vi "Parse State Queue++.vi"(0 "State Queue":string, 1 "Name (\"\" to Use UUID)":string, 2 "Response Arguments":string, 7 "Previous Error":errorcluster, 9 "Dequeue (1 ms)":i32=1, 11 "Response Timeout (-2 Use Global Settings)":i32=-2, 12 "Allowed Messages (Empty for All)":string[](array[string])) -> (3 "Name Used":string, 4 "Remaining States":string, 6 "Current State":string, 8 "Arguments":string, 10 ">> Response Source Message >>":T1, 15 ">> Source CSM >>":string)   [LabVIEW 2017, in "Communicable State Machine.lvlib"]
doc: "### Parse State Queue++.vi\n\nParses the CSM state queue and returns the next current state to be executed, along with parameters and other information.\n\n<b>Controls</b>\n- <b>State Queue</b>: The entire state queue is connected to this input. This should come from the CSM's shift register.\n- <b>Previous Error</b>: The error cluster from the CSM is connected to this input. If an error occurs and appears at this input, the current state output will return the \"Error Handler\" state.\n- <b>Name (\"\" to use uuid)</b>: CSM module name.\n- <b>Response Timeout(-2 using Global Settings)</b>: Response timeout setting for synchronous calls, If -2 is specified, the global setting will be used. You can use \"CSM - Set TMO of Sync-Reply.vi\" to change the global setting.\n- <b>Dequeue Timeout (0ms)</b>: Timeout setting for checking the CSM message queue, default is 0, meaning no wait.\n- <b>Response Arguments</b>: Response parameters from the previous state. It should be connected to the CSM's shift register to pass return values from external calls.\n\n<b>Indicators</b>\n- <b>Remaining States</b>: All concatenated states and parameters.\n- <b>Arguments</b>: Returns any parameters that may be used in the current state string. These parameters are located after the \">>\" character. <b>Note:</b> Argument variables must not contain any non-printable characters, such as newline or carriage return.\n- <b>Current State</b>: The next current state to be executed.\n- <b>Name Used</b>: The actual name assigned to this CSM module.\n- <b>Argument - State</b>: If it is a built-in state defined by CSM, this parameter indicates the previous state of this state.\n- <b>From Who</b>: If <b>Current State</b> is sent by an external source, this is the source CSM module name."
uses:
  Communicable State Machine.lvlib
  _Support/Typedef/_CSM_Response Source Message.ctl
  _Support/Typedef/_CSM_GlobalLog_MSG.ctl
  _Support/Typedef/_CSM_GlobalLog_MSG_TYPE.ctl
  _Support/Typedef/_CSM_MSG_TYPE.ctl
  _Support/Typedef/_CSM Status Change Event Data.ctl
  _Support/CSMQ/_CSMObj-Message Check.vi
  _Support/CSMQ/_CSMObj-Enqueue Cross-Module Message.vi
  _Support/CSMQ/_CSMOFGV Get.vi
  _Support/GlobalEvent/GEvt-Generate with Rule Check.vi
  _Support/FGV-BroadcastRegistry/Cache-Broadcast Registry Search Result.vi
  _Support/Common/Hex Str to U8 Data.vi
  AdvanceAPI/CSM - Revert Arguments-Safe String.vi
  AdvanceAPI/CSM - Make String Arguments Safe.vi
  _Support/Common/U8 Data to Hex Str.vi
  _Support/Priority Queue/Dequeue Element.vi
  _Support/GlobalEvent/GEvt-Convert Filter Rules - v1.0.vi
  _Support/ChangeFlag/FlagInstance-GEvt Filter.vi
  _Shared/CSM - System States.vi
  _Support/Priority Queue/Enqueue Element.vi
  _Support/ChangeFlag/FlagInstance-CSMQ FGV.vi
  _Support/ChangeFlag/FlagInstance-Broadcast Cache.vi
  AdvanceAPI/CSM - Keywords.vi
  _Support/ChangeFlag/ChangeFlag-Read.vi
  _Support/GlobalEvent/LogFilter/LogFilter - Check.vi
  _Support/CSMQ/_CSMOFGV(lvlibp).vi
  _Support/FGV-BroadcastRegistry/FGV-BroadcastRegistry(lvlibp).vi
  AdvanceAPI/CSM - List Modules.vi
  _Support/BroadcastRegistry/HelperVI/Broadcast Item Key.vi
  _Shared/Trim Single-line Text.vi
  _Support/ChangeFlag/ChangeFlagDB.vi
  _Support/CSMKVMap/CSMKVMap-Read.vi
  _Support/Error/CSM Not Allowed Message.vi
  _Support/CSMQ/_CSMObj-Add Internal Registry Rule.vi
  _Support/Message/Parse Unregister Message.vi
  _Support/Message/Parse Register Message.vi
  _Shared/Concatenate State with Arguments.vi
  _Support/Error/CSM Missing Return State Error.vi
  Utility/Build Internal State String.vi
  _Shared/Concatenate PostPostMsg Message.vi
  _Support/GlobalEvent/LogFilter/SettingVIs/Set CSM StateType Filter.vi
  _Support/GlobalEvent/LogFilter/SettingVIs/Set Global StateType Filter.vi
  _Support/GlobalEvent/LogFilter/SettingVIs/Set CSM State Filter.vi
  _Support/GlobalEvent/LogFilter/SettingVIs/Set CSM LogType Filter.vi
  _Support/GlobalEvent/LogFilter/SettingVIs/Set Global State Filter.vi
  _Support/GlobalEvent/LogFilter/SettingVIs/Set Global LogType Filter.vi
  _Support/GlobalEvent/LogFilter/SettingVIs/Set Global CSM Filter.vi
  _Support/GlobalEvent/FGV-GEvt Filter Rules(lvlibp).vi
  _Support/GlobalEvent/LogFilter/LogFilter.lvclass
  _Shared/CSM Shared.lvlib
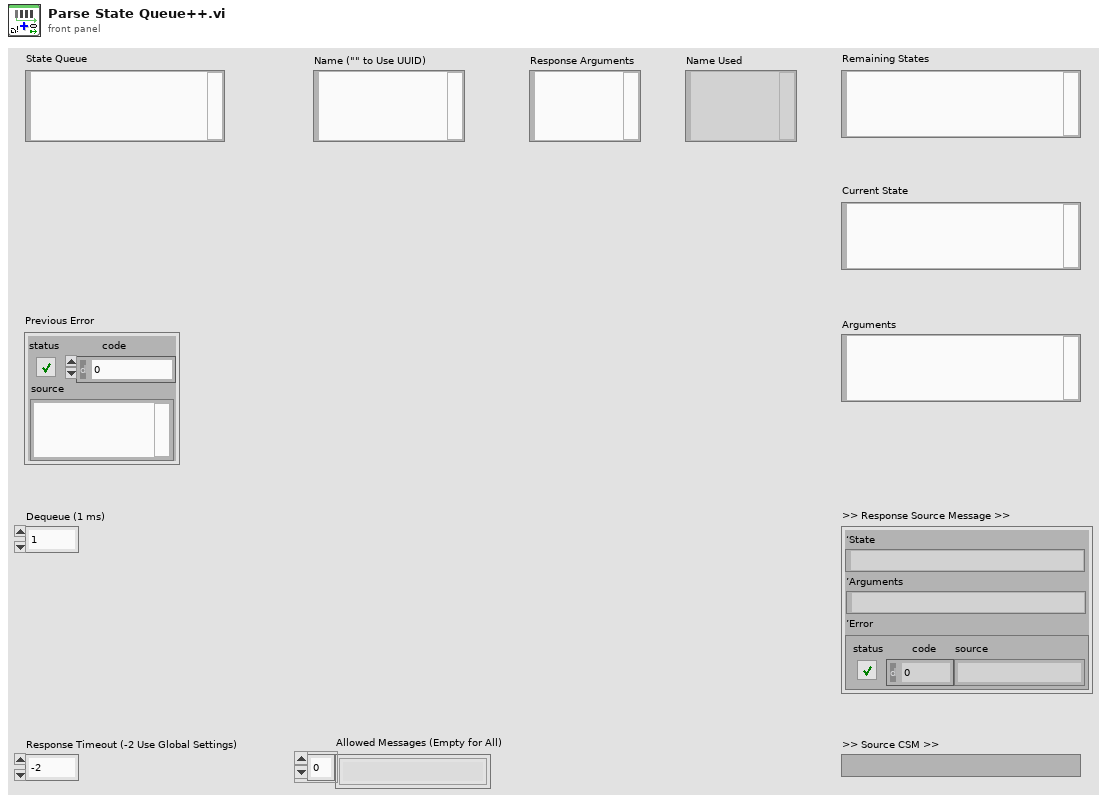
[diagram p1: front panel]
types:
  T1 = typedef "Communicable State Machine.lvlib/_CSM_Response Source Message.ctl" = cluster{"‘State":string, "’Arguments":string, "’Error":errorcluster}
  T2 = typedef "Communicable State Machine.lvlib/_CSM_GlobalLog_MSG.ctl" = cluster{"Name (\"\" to Use UUID)":string, "Current State":string, "Arguments":string, "Source Message":T1, "Source Module":string, "Complete(T)/Start(F)":bool, "LogType":T3, "Time Stamp":timestamp}
  T3 = typedef "Communicable State Machine.lvlib/_CSM_GlobalLog_MSG_TYPE.ctl" = enum16{"User Log", "State Change", "Status", "Interrupt", "Register", "Unregister", "Error Log", "Module Created", "Module Destroyed"}
  T4 = typedef "Communicable State Machine.lvlib/GEvt-Refs.ctl" = cluster{"Event":refnum<user-event>, "Queues":refnum<queue>[], "Valid":bool}
  T5 = typedef "Communicable State Machine.lvlib/_CSMObj.ctl" = cluster{"info":T6, "Refs":T8}
  T6 = typedef "Communicable State Machine.lvlib/_CSMObj-Info.ctl" = cluster{"Module Name":string, "Requested Name":string, "Group Name":string, "Mode":T7, "Allowed Messages":string[]}
  T7 = typedef "Communicable State Machine.lvlib/_CSM_MODE.ctl" = enum16{"Not Exist", "Stand Alone", "CSM", "Worker", "Worker Agent", "Chain Node", "Chain"}
  T8 = typedef "Communicable State Machine.lvlib/_CSMObj-Refs.ctl" = cluster{"WatchDogQ":refnum<queue>, "CSMDataDVR":refnum<data-value>, "Queue":T9, "GroupDataDVR":refnum<data-value>, "TagMap":refnum<data-value>, "ExitEvent":refnum<user-event>, "NewStateEvent":refnum<user-event>, "StatusChangeEvent":refnum<user-event>}
  T9 = typedef "Communicable State Machine.lvlib/Priority Queue.ctl" = cluster{"HPriorityQ":refnum<queue>, "LowPriorityQ":refnum<queue>}
  T10 = typedef "Communicable State Machine.lvlib/_CSM_MSG_TYPE.ctl" = enum16{"Sync Message(-@)", "Async Message(->)", "Async without Response(->|)", "Async Response", "Broadcast(-><all>)", "Broadcast(-><status>)", "Broadcast(-><interrupt>)", "Append to JKISM States", "Append to JKISM States(High Priority)", "Broadcast(-><state>)"}
  T11 = typedef "Communicable State Machine.lvlib/_CSM Status Change Event Data.ctl" = cluster{"ModuleName":string, "Status":string, "Arguments":string}
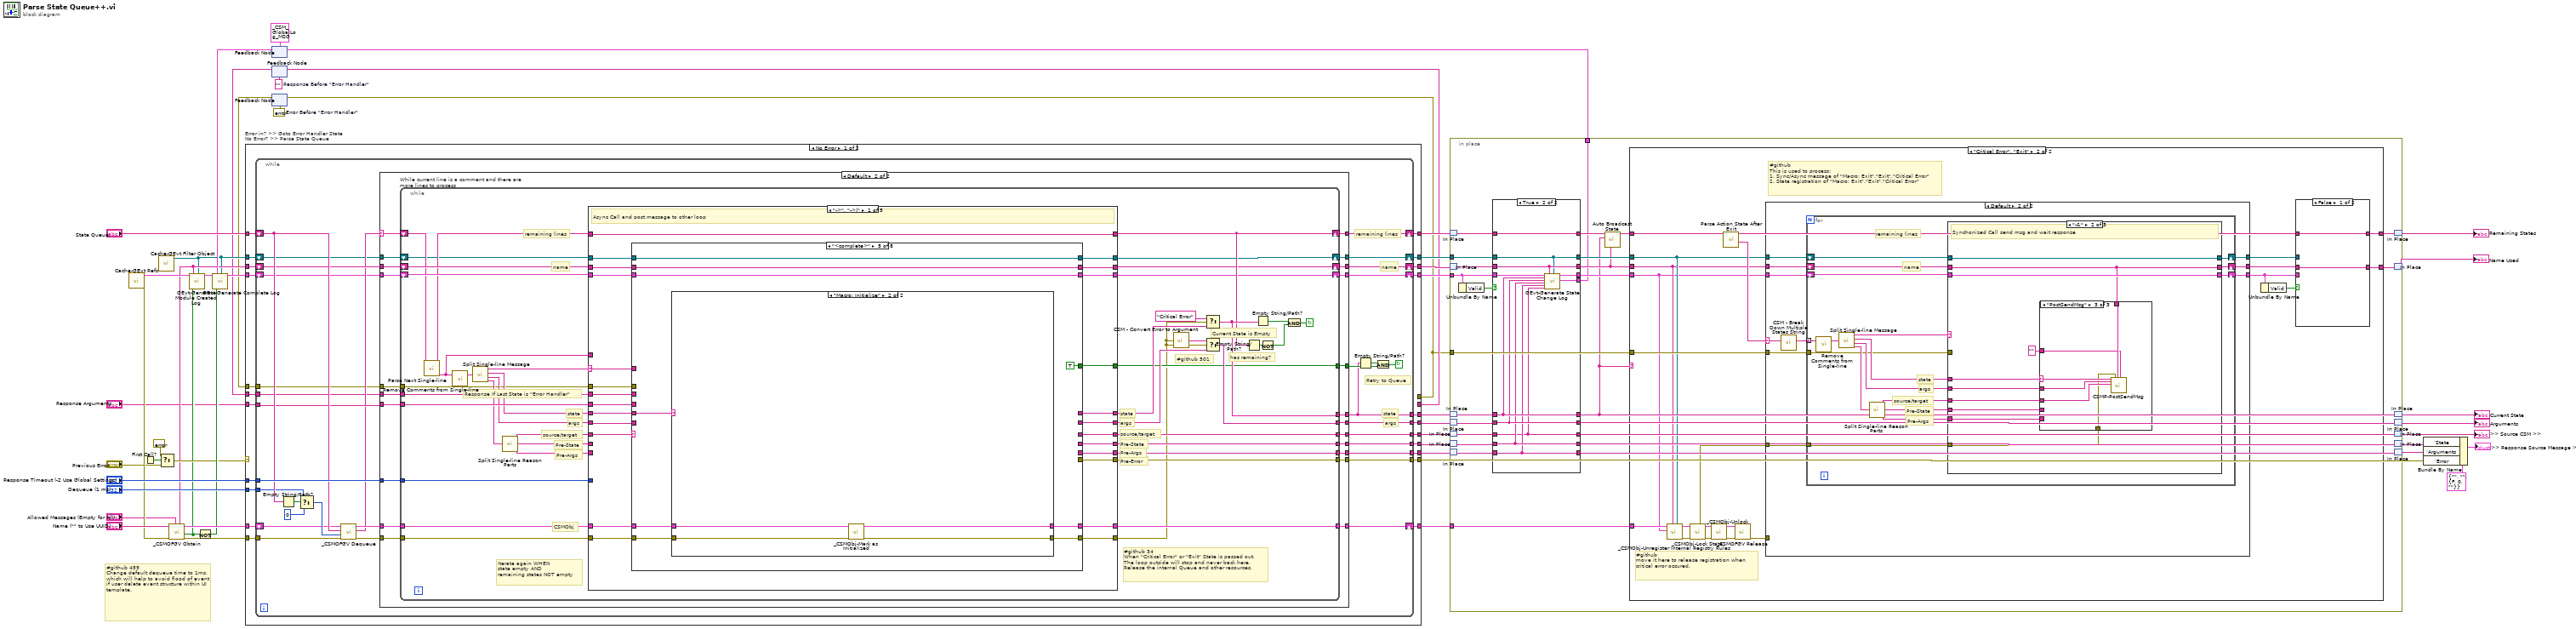
[diagram p0: block diagram]
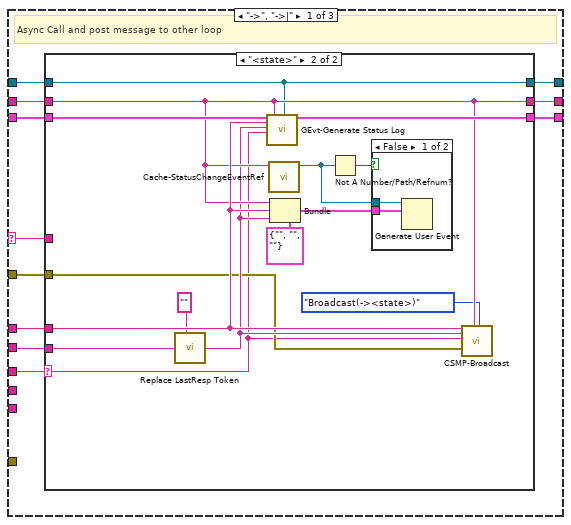
[diagram p4: hidden frame]
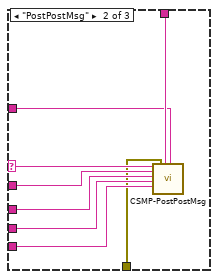
[diagram p8: hidden frame]
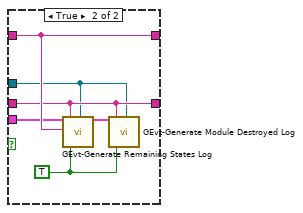
[diagram p10: hidden frame]
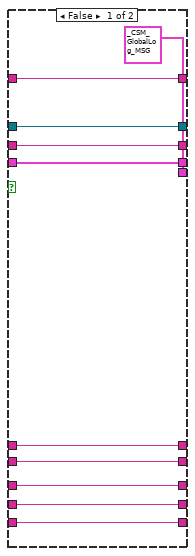
[diagram p11: hidden frame]
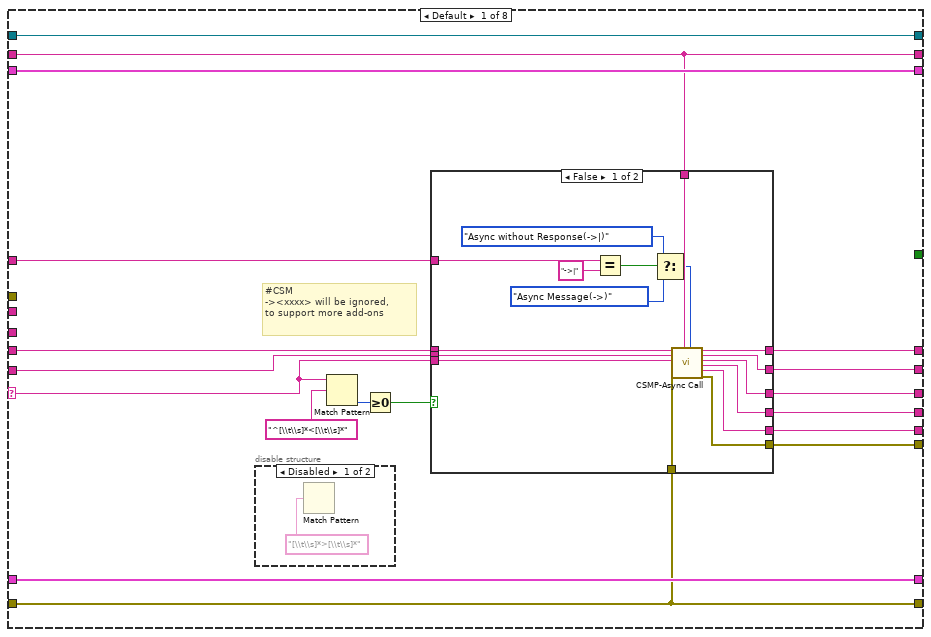
[diagram p13: hidden frame]
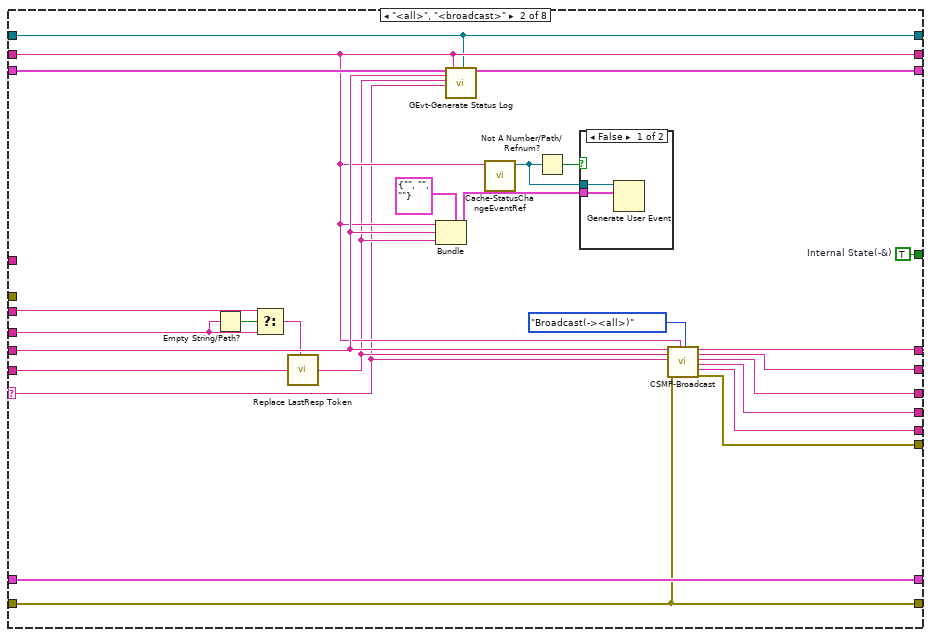
[diagram p16: hidden frame]
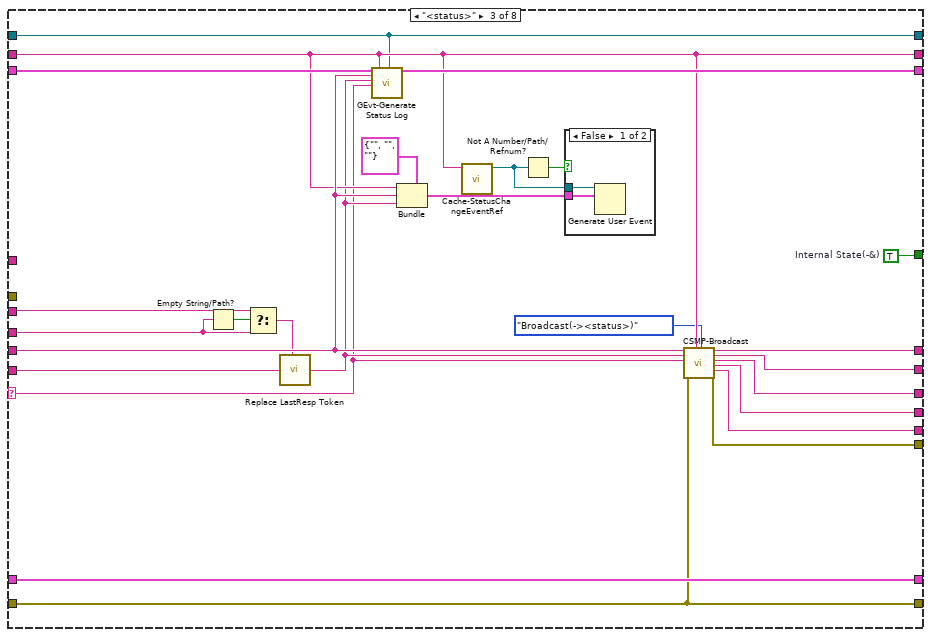
[diagram p18: hidden frame]
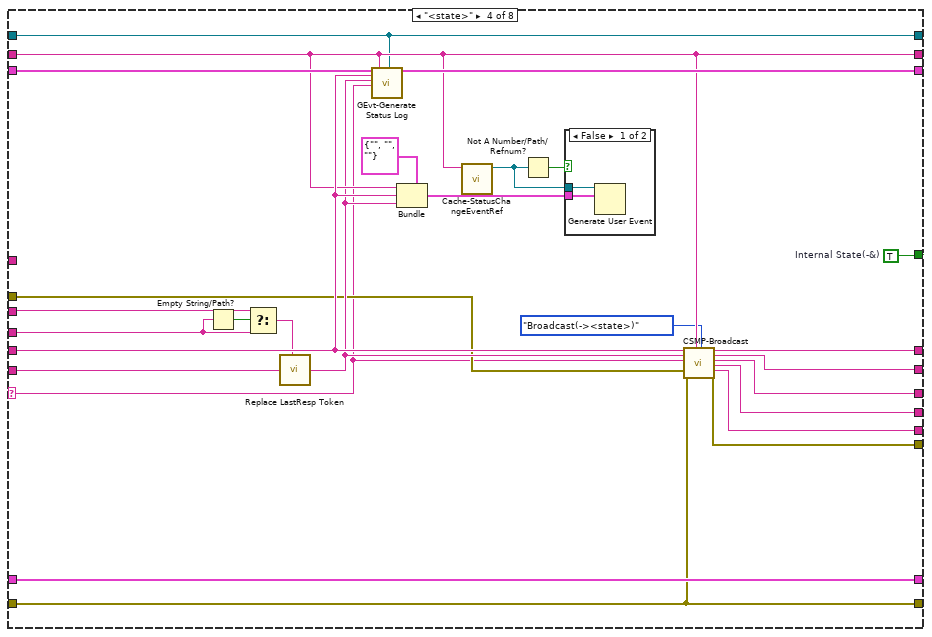
[diagram p20: hidden frame]
diagram:
  w4 = errorcluster {"status"=FALSE, "code"=0, "source"=""}  # Error Before "Error Handler"
  w7 = ""  # Response Before "Error Handler"
  # "#github 459\nChange default dequeue time to 1ms, which will help to avoid flood of event\nif user delete event structure within UI template."
  n1 = call "Cache-GEvt Refs.vi"() -> ("error out"=w33:errorcluster, "CSM Global Log Ref"=w14:T4)  [unwired: 10 in]
  n2 = First Call?() -> (First Call?: T/F=w18:bool)
  n3 = call "Cache-GEvt Filter Object.vi"() -> ("CSM:LogFilter.lvclass"=w9:refnum<class "LogFilter.lvclass">)  [unwired: 11 in]
  n4 = Select(t=errorcluster {"status"=FALSE, "code"=0, "source"=""}, s=w18, f="Previous Error") -> (s? t:f=w16:errorcluster)
  n5 = call "_CSMOFGV Obtain.vi"("Allowed Messages (Empty For All)"="Allowed Messages (Empty for All)", "Error In"=w33, "Name (\"\" to Use UUID) In"="Name (\"\" to Use UUID)") -> ("error out"=w46:errorcluster, "Create? (T)/Cached(F)"=w11:bool, "CSM-Obj"=w45:T5, "Name"=w12:string)  [unwired: 5 in]
  n6 = call "GEvt-Generate Module Created Log.vi"("CSM Global Log Event"=w14, "Name (\"\" to Use UUID)"=w12, "Created?"=w11, "CSM:LogFilter.lvclass"=w9) -> ("CSM Global Log Event Out"=w13:T4)  [unwired: 14 in, 1 out]
  n7 = Not(x=w11) -> (.not. x?=w19:bool)
  n8 = feedback #1(T2 {"Name (\"\" to Use UUID)"="", "Current State"="", "Arguments"="", "Source Message"={"‘State"="", "’Arguments"="", "’Error"={"status"=FALSE, "code"=0, "source"=""}}, "Source Module"="", "Complete(T)/Start(F)"=FALSE, "LogType"=enum."State Change", "Time Stamp"=timestamp(0 s since 1904-01-01)} ("event data")) -> (w24:T2)
  n9 = call "GEvt-Generate Complete Log.vi"("CSM Global Log Event"=w13, "Event Data"=w24, "Enable?"=w19, "CSM:LogFilter.lvclass"=w9) -> ("CSM Global Log Event Out"=w23:T4)  [unwired: 15 in]
  n10 = feedback #2(w7) -> (w5:string)
  n11 = feedback #3(w4) -> (w3:errorcluster)
  n12 = case "Error in? >> Goto Error Handler State\nNo Error? >> Parse State Queue" shown="No Error" w16 {
    selector: w16 -> [_ w582]
    tunnel: [w69 w591] -> w36
    tunnel: [w71 "Error Handler"] -> w44
    tunnel: [w70 w587] -> w43
    tunnel: "State Queue" -> [w66 w591]
    tunnel: "Response Timeout (-2 Use Global Settings)" -> [w68 _]
    tunnel: w45 -> [w61 w586]
    tunnel: [w67 _] -> w41
    tunnel: "Dequeue (1 ms)" -> [w65 _]
    tunnel: [w64 _] -> w42
    tunnel: "Response Arguments" -> [w63 w583]
    tunnel: w46 -> [w62 w585]
    tunnel: w12 -> [w60 w589]
    tunnel: w23 -> [w59 w588]
    tunnel: [w58 w589] -> w32
    tunnel: [w57 w588] -> w31
    tunnel: [w56 _] -> w27
    tunnel: [w55 _] -> w21
    tunnel: w9 -> [w54 w584]
    tunnel: [w53 w584] -> w10
    tunnel: [_ w583] -> w6
    tunnel: w5 -> [w52 _]
    tunnel: [_ w582] -> w2
    tunnel: w3 -> [w51 _]
    tunnel: [w50 w581] -> w1
    frame No Error {
      n13 = while {
        tunnel: [w102] -> w70
        tunnel: w68 -> [w100]
        tunnel: [w99] -> w67
        tunnel: w65 -> [w95]
        tunnel: w62 -> [w90]
        shift-right: [w101] -> w69
        shift-left: w66 -> [w96]
        tunnel: w63 -> [w91]
        tunnel: [w83] -> w71
        tunnel: [w92] -> w64
        shift-right: [w80] -> w58
        shift-left: w60 -> [w88]
        shift-right: [w79] -> w57
        shift-left: w59 -> [w81]
        tunnel: [w78] -> w56
        tunnel: [w77] -> w55
        shift-right: [w75] -> w53
        shift-left: w54 -> [w76]
        tunnel: w52 -> [w74]
        tunnel: w51 -> [w73]
        shift-right: [w72] -> w50
        shift-left: w61 -> [w89]
        stop <- w85 continue-if-true
        # "args"
        # "state"
        # "name"
        # "remaining lines"
        # "Retry to Queue"
        n14 = Empty String/Path?(string/path=w96) -> (empty?=w97:bool)
        n15 = Select(t=w95, s=w97, f=0) -> (s? t:f=w93:i32)
        n16 = call "_CSMOFGV Dequeue.vi"("Error In"=w90, "Dequeue Timeout (0ms)"=w93, "State (S) In (\"\")"=w96, "CSMQ In"=w89) -> ("error out"=w86:errorcluster, "States Out"=w87:string, "CSMQ Out"=w98:T5)  [unwired: 5 in]
        n17 = case shown="Default" w87 {
          selector: w87 -> [_ w122]
          tunnel: [_ w128] -> w83
          tunnel: [_ w127] -> w102
          tunnel: [_ w126] -> w101
          tunnel: w100 -> [_ w125]
          tunnel: [_ w124] -> w99
          tunnel: w88 -> [w106 w123]
          tunnel: w98 -> [w103 w121]
          tunnel: w86 -> [_ w120]
          tunnel: [_ w119] -> w92
          tunnel: w91 -> [_ w118]
          tunnel: [_ w117] -> w84
          tunnel: w81 -> [w105 w116]
          tunnel: [w106 w115] -> w80
          tunnel: [w105 w114] -> w79
          tunnel: [_ w113] -> w78
          tunnel: [_ w112] -> w77
          tunnel: w76 -> [w104 w111]
          tunnel: [w104 w110] -> w75
          tunnel: w74 -> [_ w109]
          tunnel: w73 -> [_ w108]
          tunnel: [w103 w107] -> w72
          frame "" {
            # "Dispatch Mode\n1. Error will Occurred\n2. Add Macro: Exit\n3. The Queue will regenerated\n4. But it will go Through Macro: Exit\n5. After Exit(queue released), then another Worker will be triggered."
            # "Do Nothing if Empty String"
            # "<< Wiring into the Case Selector is much more performant than using \"Empty String/Path?\" primitive"
          }
          frame Default {
            n18 = while "While current line is a comment and there are more lines to process" {
              tunnel: [w157] -> w128
              tunnel: [w159] -> w127
              shift-right: [w153] -> w126
              shift-left: w122 -> [w145]
              tunnel: w125 -> [w166]
              tunnel: [w158] -> w124
              tunnel: w121 -> [w165]
              tunnel: w120 -> [w162]
              tunnel: [w164] -> w119
              tunnel: w118 -> [w163]
              tunnel: [w155] -> w117
              shift-right: [w134] -> w115
              shift-left: w123 -> [w152]
              shift-right: [w132] -> w114
              shift-left: w116 -> [w151]
              tunnel: [w150] -> w113
              tunnel: [w139] -> w112
              shift-right: [w133] -> w110
              shift-left: w111 -> [w135]
              tunnel: w109 -> [w137]
              tunnel: w108 -> [w136]
              tunnel: [w131] -> w107
              stop <- w154 continue-if-true
              # "#github 501"
              # "Response If Last State is \"Error Handler\""
              # "source/target"
              # "Pre-Error"
              # "args"
              # "state"
              # "Pre-Args"
              # "Pre-State"
              # "source/target"
              # "Pre-Args"
              # "Pre-State"
              # "CSMObj"
              # "#github 34\nWhen \"Critical Error\" or \"Exit\" State is passed out,\nThe loop outside will stop and never back here.\nRelease the internal Queue and other resources."
              # "name"
              # "remaining lines"
              # "Iterate again WHEN\nstate empty AND\nremaining states NOT empty"
              # "args"
              # "state"
              # "Current State is Empty"
              # "has remaining?"
              n19 = call "Parse Next Single-line.vi"("States Queue"=w145) -> ("Next Single-line State"=w138:string, "Remaining States Queue"=w144:string)  [unwired: 9 in]
              n20 = call "Remove Comments from Single-line.vi"("single-line text"=w138) -> ("single-line text without comments"=w149:string)  [unwired: 2 in]
              n21 = call "Split Single-line Message.vi"("single-line text"=w149) -> ("operator"=w146:string, "state"=w147:string, "args"=w148:string, "source/target"=w143:string)  [unwired: 6 in]
              n22 = call "Split Single-line Reason Parts.vi"("Single-line -& Reason"=w143) -> ("CSM Name"=w142:string, "`State"=w141:string, "`Arguments"=w140:string)  [unwired: 12 in]
              n23 = case shown="\"->\", \"->|\"" w146 {
                selector: w146 -> [w183 _ _ _ _]
                tunnel: w147 -> [w191 w407 w434 w491 w580]
                tunnel: w148 -> [w190 w406 w436 w490 w579]
                tunnel: [w194 w404 w438 w489 w580] -> w161
                tunnel: [w193 w403 w437 w488 w579] -> w160
                tunnel: w152 -> [w189 w408 w427 w483 w573]
                tunnel: w142 -> [w192 w405 w426 w486 w576]
                tunnel: w166 -> [_ w397 _ _ _]
                tunnel: w165 -> [w181 w411 w421 w497 w577]
                tunnel: w144 -> [w184 w410 w430 w493 w575]
                tunnel: [w188 w401 w433 w485 _] -> w164
                tunnel: w163 -> [w186 _ w415 _ _]
                tunnel: w162 -> [w187 w398 w420 w496 w578]
                tunnel: [w174 w398 w435 w495 w578] -> w130
                tunnel: [w176 w402 w423 w487 w576] -> w158
                tunnel: [w182 w411 w432 w494 w577] -> w131
                tunnel: [w185 _ w431 w481 _] -> w155
                tunnel: [w184 w410 w430 w492 w575] -> w153
                tunnel: w151 -> [w180 w409 w429 w482 w574]
                tunnel: [w179 w409 w429 w482 w574] -> w132
                tunnel: [w177 w400 w428 w476 _] -> w150
                tunnel: [w178 w408 w427 w483 w573] -> w134
                tunnel: w141 -> [_ _ w425 w484 _]
                tunnel: w140 -> [_ _ w424 w477 _]
                tunnel: [w175 w399 w422 w475 _] -> w139
                tunnel: w135 -> [w173 w396 w412 w474 w572]
                tunnel: w138 -> [_ _ _ w480 _]
                tunnel: w137 -> [w172 _ w414 _ _]
                tunnel: w136 -> [w171 _ _ _ _]
                tunnel: [w170 w396 w412 w474 w572] -> w133
                frame "->", "->|" {
                  # "Async Call and post message to other loop"
                  n24 = case shown="\"<complete>\"" w192 {
                    selector: w192 -> [w198 w235 w263 w291 _ w346 w376 w393]
                    tunnel: [w206 w241 w276 w307 _ w345 w375 w392] -> w194
                    tunnel: [w205 w242 w273 w304 _ w344 w374 w391] -> w193
                    tunnel: w191 -> [w212 w251 w277 w308 w320 w348 w364 w381]
                    tunnel: w190 -> [w207 w250 w274 w305 _ w347 w363 w380]
                    tunnel: w189 -> [w208 w249 w275 w306 w326 w350 w365 w382]
                    tunnel: [w204 w244 w271 w302 _ w342 w372 w389] -> w188
                    tunnel: w187 -> [w200 w247 w279 w293 w322 w349 w377 w394]
                    tunnel: w186 -> [_ w237 w266 w297 _ w336 _ _]
                    tunnel: [_ w259 w287 w316 TRUE ("Internal State(-&)") w359 w378 w395] -> w185
                    tunnel: w183 -> [w211 _ _ _ _ _ _ _]
                    tunnel: [w210 w255 w286 w294 w324 w355 w368 w385] -> w182
                    tunnel: w181 -> [w210 w255 w286 w294 w323 w355 w369 w386]
                    tunnel: [w209 w253 w280 w310 w327 w352 w366 w383] -> w179
                    tunnel: w180 -> [w209 w252 w281 w311 w327 w353 w367 w384]
                    tunnel: [w208 w249 w275 w306 w326 w350 w365 w382] -> w178
                    tunnel: [w203 w245 w270 w301 _ w341 w371 w388] -> w177
                    tunnel: [w202 w243 w272 w303 _ w343 w373 w390] -> w176
                    tunnel: [w201 w246 w278 w309 _ w340 w370 w387] -> w175
                    tunnel: [w200 w247 w279 w293 w321 w349 w377 w394] -> w174
                    tunnel: w173 -> [w195 w234 w262 w290 w319 w334 w362 w379]
                    tunnel: w172 -> [_ w238 w265 w296 _ w337 _ _]
                    tunnel: w171 -> [_ _ _ w292 _ _ _ _]
                    tunnel: [w195 w234 w262 w290 w319 w334 w362 w379] -> w170
                    frame Default {
                      # "#CSM\n-><xxxx> will be ignored,\nto support more add-ons"
                      n25 = disable-structure shown="Disabled" {
                        frame Disabled {
                          n26 = Match Pattern(regular expression="[\\t\\s]*>[\\t\\s]*") -> ()  [unwired: 2 in, 4 out]
                        }
                        frame Enabled {
                        }
                      }
                      n27 = Match Pattern(string=w198, regular expression="^[\\t\\s]*<[\\t\\s]*") -> (offset past match=w197:i32)  [unwired: 1 in, 3 out]
                      n28 = Greater Or Equal To 0?(x=w197) -> (x >= 0?=w196:bool)
                      n29 = case shown="False" w196 {
                        tunnel: w212 -> [w230 w233]
                        tunnel: w211 -> [w229 _]
                        tunnel: w208 -> [w228 _]
                        tunnel: w207 -> [w227 w232]
                        tunnel: [w222 w233] -> w206
                        tunnel: [w221 w232] -> w205
                        tunnel: [w220 _] -> w204
                        tunnel: [w219 _] -> w203
                        tunnel: [w218 w231] -> w202
                        tunnel: [w217 _] -> w201
                        tunnel: w200 -> [w215 _]
                        tunnel: w198 -> [w214 w231]
                        frame False {
                          n30 = Equal?(x=w229, y="->|") -> (x = y?=w225:bool)
                          n31 = Select(t=_CSM_MSG_TYPE."Async without Response(->|)" ("Msg Type"), s=w225, f=_CSM_MSG_TYPE."Async Message(->)" ("Msg Type")) -> (s? t:f=w216:T10)
                          n32 = call "CSMP-Async Call.vi"("State"=w230, "Args"=w227, "Source/target"=w214, "Error In"=w215, "Module Name"=w228, "Msg Type"=w216) -> ("State Out"=w222:string, "Args Out"=w221:string, "Source/target Out"=w218:string, "Pre-State Out"=w220:string, "Pre-Args Out"=w219:string, "Error"=w217:errorcluster)  [unwired: 8 in]
                        }
                        frame True {
                        }
                      }
                    }
                    frame "<all>", "<broadcast>" {
                      w259 = TRUE  # Internal State(-&)
                      n33 = Empty String/Path?(string/path=w237) -> (empty?=w239:bool)
                      n34 = Select(t=w238, s=w239, f=w237) -> (s? t:f=w236:string)
                      n35 = call "Replace LastResp Token.vi"("LastResp"=w236, "Argument"=w250) -> ("Argument Out"=w240:string)  [unwired: 5 in]
                      n36 = Bundle(cluster=T11 {"ModuleName"="", "Status"="", "Arguments"=""} ("event data"), "ModuleName"=w249, "Status"=w251, "Arguments"=w240) -> (w256:T11)
                      n37 = call "GEvt-Generate Status Log.vi"("CSM Global Log Event"=w252, "Current State"=w251, "Arguments"=w240, "Source Module"=w235, "Name (\"\" to Use UUID)"=w249, "CSM:LogFilter.lvclass"=w234) -> ("CSM Global Log Event Out"=w253:T4)  [unwired: 12 in, 1 out]
                      n38 = call "Cache-StatusChangeEventRef.vi"("Name (\"\" to Use UUID) In"=w249) -> ("Status Change Event"=w254:refnum<user-event>)  [unwired: 9 in, 1 out]
                      n39 = Not A Number/Path/Refnum?(number/path/refnum=w254) -> (NaN/Path/Refnum?=w258:bool)
                      n40 = case shown="False" w258 {
                        tunnel: w254 -> [w261 _]
                        tunnel: w256 -> [w260 _]
                        frame False {
                          n41 = Generate User Event(user event=w261, event data cluster=w260) -> ()  [unwired: 2 in, 2 out]
                        }
                        frame True {
                        }
                      }
                      n42 = call "CSMP-Broadcast.vi"("State"=w251, "Args"=w240, "Source/target"=w235, "Error In"=w247, "Module Name"=w249, "Msg Type"=_CSM_MSG_TYPE."Broadcast(-><all>)") -> ("State Out"=w241:string, "Args Out"=w242:string, "Source/target Out"=w243:string, "Pre-State Out"=w244:string, "Pre-Args Out"=w245:string, "Error"=w246:errorcluster)  [unwired: 8 in]
                    }
                    frame "<status>" {
                      w287 = TRUE  # Internal State(-&)
                      n43 = Empty String/Path?(string/path=w266) -> (empty?=w267:bool)
                      n44 = Select(t=w265, s=w267, f=w266) -> (s? t:f=w264:string)
                      n45 = call "Replace LastResp Token.vi"("LastResp"=w264, "Argument"=w274) -> ("Argument Out"=w268:string)  [unwired: 5 in]
                      n46 = call "GEvt-Generate Status Log.vi"("CSM Global Log Event"=w281, "Current State"=w277, "Arguments"=w268, "Source Module"=w263, "Name (\"\" to Use UUID)"=w275, "CSM:LogFilter.lvclass"=w262) -> ("CSM Global Log Event Out"=w280:T4)  [unwired: 12 in, 1 out]
                      n47 = Bundle(cluster=T11 {"ModuleName"="", "Status"="", "Arguments"=""} ("event data"), "ModuleName"=w275, "Status"=w277, "Arguments"=w268) -> (w283:T11)
                      n48 = call "Cache-StatusChangeEventRef.vi"("Name (\"\" to Use UUID) In"=w275) -> ("Status Change Event"=w282:refnum<user-event>)  [unwired: 9 in, 1 out]
                      n49 = Not A Number/Path/Refnum?(number/path/refnum=w282) -> (NaN/Path/Refnum?=w285:bool)
                      n50 = case shown="False" w285 {
                        tunnel: w282 -> [w289 _]
                        tunnel: w283 -> [w288 _]
                        frame False {
                          n51 = Generate User Event(user event=w289, event data cluster=w288) -> ()  [unwired: 2 in, 2 out]
                        }
                        frame True {
                        }
                      }
                      n52 = call "CSMP-Broadcast.vi"("State"=w277, "Args"=w268, "Source/target"=w263, "Error In"=w279, "Module Name"=w275, "Msg Type"=_CSM_MSG_TYPE."Broadcast(-><status>)") -> ("State Out"=w276:string, "Args Out"=w273:string, "Source/target Out"=w272:string, "Pre-State Out"=w271:string, "Pre-Args Out"=w270:string, "Error"=w278:errorcluster)  [unwired: 8 in]
                    }
                    frame "<state>" {
                      w316 = TRUE  # Internal State(-&)
                      n53 = Empty String/Path?(string/path=w297) -> (empty?=w298:bool)
                      n54 = Select(t=w296, s=w298, f=w297) -> (s? t:f=w295:string)
                      n55 = call "Replace LastResp Token.vi"("LastResp"=w295, "Argument"=w305) -> ("Argument Out"=w299:string)  [unwired: 5 in]
                      n56 = call "GEvt-Generate Status Log.vi"("CSM Global Log Event"=w311, "Current State"=w308, "Arguments"=w299, "Source Module"=w291, "Name (\"\" to Use UUID)"=w306, "CSM:LogFilter.lvclass"=w290) -> ("CSM Global Log Event Out"=w310:T4)  [unwired: 12 in, 1 out]
                      n57 = Bundle(cluster=T11 {"ModuleName"="", "Status"="", "Arguments"=""} ("event data"), "ModuleName"=w306, "Status"=w308, "Arguments"=w299) -> (w313:T11)
                      n58 = call "Cache-StatusChangeEventRef.vi"("Name (\"\" to Use UUID) In"=w306) -> ("Status Change Event"=w312:refnum<user-event>)  [unwired: 9 in, 1 out]
                      n59 = Not A Number/Path/Refnum?(number/path/refnum=w312) -> (NaN/Path/Refnum?=w315:bool)
                      n60 = case shown="False" w315 {
                        tunnel: w312 -> [w318 _]
                        tunnel: w313 -> [w317 _]
                        frame False {
                          n61 = Generate User Event(user event=w318, event data cluster=w317) -> ()  [unwired: 2 in, 2 out]
                        }
                        frame True {
                        }
                      }
                      n62 = call "CSMP-Broadcast.vi"("State"=w308, "Args"=w299, "Source/target"=w291, "Response For Message.’Error"=w292, "Error In"=w293, "Module Name"=w306, "Msg Type"=_CSM_MSG_TYPE."Broadcast(-><state>)") -> ("State Out"=w307:string, "Args Out"=w304:string, "Source/target Out"=w303:string, "Pre-State Out"=w302:string, "Pre-Args Out"=w301:string, "Error"=w309:errorcluster)  [unwired: 7 in]
                    }
                    frame "<complete>" {
                      n63 = case shown="\"Macro: Initialize\"" w320 {
                        tunnel: [w329 w330] -> w324
                        tunnel: w323 -> [w329 w331]
                        tunnel: w322 -> [w328 w333]
                        tunnel: [w328 w332] -> w321
                        frame Default {
                        }
                        frame "Macro: Initialize" {
                          n64 = call "_CSMObj-Mark as Initialized.vi"("Error In"=w333, "CSMQ In"=w331) -> ("error out"=w332:errorcluster, "CSMQ Out"=w330:T5)  [unwired: 8 in]
                        }
                      }
                    }
                    frame "<interput>", "<interrupt>", "<interupt>" {
                      w359 = TRUE  # Internal State(-&)
                      # "for typo"
                      n65 = Empty String/Path?(string/path=w336) -> (empty?=w338:bool)
                      n66 = Select(t=w337, s=w338, f=w336) -> (s? t:f=w335:string)
                      n67 = call "Replace LastResp Token.vi"("LastResp"=w335, "Argument"=w347) -> ("Argument Out"=w339:string)  [unwired: 5 in]
                      n68 = call "GEvt-Generate Interrupt Log.vi"("CSM Global Log Event"=w353, "Current State"=w348, "Arguments"=w339, "Name (\"\" to Use UUID)"=w350, "CSM:LogFilter.lvclass"=w334) -> ("CSM Global Log Event Out"=w352:T4)  [unwired: 13 in, 1 out]
                      n69 = Bundle(cluster=T11 {"ModuleName"="", "Status"="", "Arguments"=""} ("event data"), "ModuleName"=w350, "Status"=w348, "Arguments"=w339) -> (w356:T11)
                      n70 = call "Cache-StatusChangeEventRef.vi"("Name (\"\" to Use UUID) In"=w350) -> ("Status Change Event"=w354:refnum<user-event>)  [unwired: 9 in, 1 out]
                      n71 = Not A Number/Path/Refnum?(number/path/refnum=w354) -> (NaN/Path/Refnum?=w358:bool)
                      n72 = case shown="False" w358 {
                        tunnel: w354 -> [w361 _]
                        tunnel: w356 -> [w360 _]
                        frame False {
                          n73 = Generate User Event(user event=w361, event data cluster=w360) -> ()  [unwired: 2 in, 2 out]
                        }
                        frame True {
                        }
                      }
                      n74 = call "CSMP-Broadcast.vi"("State"=w348, "Args"=w339, "Source/target"=w346, "Error In"=w349, "Module Name"=w350, "Msg Type"=_CSM_MSG_TYPE."Broadcast(-><interrupt>)") -> ("State Out"=w345:string, "Args Out"=w344:string, "Source/target Out"=w343:string, "Pre-State Out"=w342:string, "Pre-Args Out"=w341:string, "Error"=w340:errorcluster)  [unwired: 8 in]
                    }
                    frame "<register>" {
                      w378 = TRUE  # Internal State(-&)
                      n75 = call "GEvt-Generate Register Log.vi"("CSM Global Log Event"=w367, "Current State"=w364, "Arguments"=w363, "Name (\"\" to Use UUID)"=w365, "CSM:LogFilter.lvclass"=w362) -> ("CSM Global Log Event Out"=w366:T4)  [unwired: 13 in, 1 out]
                      n76 = call "CSMP-Register Status.vi"("State"=w364, "Args"=w363, "Source/target"=w376, "Error In"=w377, "CSMQ In"=w369, "Module Name"=w365) -> ("CSMQ Out"=w368:T5, "State Out"=w375:string, "Args Out"=w374:string, "Source/target Out"=w373:string, "Pre-State Out"=w372:string, "Pre-Args Out"=w371:string, "Error"=w370:errorcluster)  [unwired: 7 in]
                    }
                    frame "<unregister>" {
                      w395 = TRUE  # Internal State(-&)
                      n77 = call "GEvt-Generate Unregister Log.vi"("CSM Global Log Event"=w384, "Current State"=w381, "Arguments"=w380, "Name (\"\" to Use UUID)"=w382, "CSM:LogFilter.lvclass"=w379) -> ("CSM Global Log Event Out"=w383:T4)  [unwired: 13 in, 1 out]
                      n78 = call "CSMP-Unregister Status.vi"("State"=w381, "Args"=w380, "Source/target"=w393, "Error In"=w394, "CSMQ In"=w386, "Module Name"=w382) -> ("CSMQ Out"=w385:T5, "State Out"=w392:string, "Args Out"=w391:string, "Source/target Out"=w390:string, "Pre-State Out"=w389:string, "Pre-Args Out"=w388:string, "Error"=w387:errorcluster)  [unwired: 7 in]
                    }
                  }
                }
                frame "-@" {
                  # "Synchonized Call send msg and wait response"
                  n79 = call "CSMP-Sync Call.vi"("State"=w407, "Args"=w406, "Source/target"=w405, "Error In"=w398, "Response Timeout (-2 Using Global Settings)"=w397, "Module Name"=w408) -> ("State Out"=w404:string, "Args Out"=w403:string, "Source/target Out"=w402:string, "Pre-State Out"=w401:string, "Pre-Args Out"=w400:string, "Error"=w399:errorcluster)  [unwired: 8 in]
                }
                frame "-&" {
                  w431 = TRUE  # Internal State(-&)
                  # "#github 413\nSend and Wait for Reply VI could not get response when error occurred in the calling state. \"Response Arguments\" is over-written by response of \"Error Handler\""
                  # "Synchonized Call send msg and wait response"
                  n80 = Empty String/Path?(string/path=w415) -> (empty?=w416:bool)
                  n81 = Select(t=w414, s=w416, f=w415) -> (s? t:f=w413:string)
                  n82 = call "_CSMObj-Lock State.vi"("Error In"=w420, "CSMQ In"=w421) -> ("error out"=w418:errorcluster, "CSMQ Out"=w419:T5, "Error"=w417:errorcluster)  [unwired: 5 in, 1 out]
                  n83 = case shown="Default" w434 {
                    selector: w434 -> [w441 w456 w470]
                    tunnel: ["Critical Error" ("before match") w447 w469] -> w438
                    tunnel: [w443 w448 w466] -> w437
                    tunnel: w426 -> [_ w454 w467]
                    tunnel: w436 -> [_ w455 w468]
                    tunnel: w413 -> [_ w457 w461]
                    tunnel: w418 -> [_ w460 w464]
                    tunnel: w427 -> [_ w458 w471]
                    tunnel: [w440 w450 w473] -> w433
                    tunnel: w425 -> [w440 w453 w473]
                    tunnel: w424 -> [w439 w452 w472]
                    tunnel: [w439 w451 w472] -> w428
                    tunnel: [_ w459 w463] -> w422
                    tunnel: [_ w449 w465] -> w423
                    tunnel: w417 -> [_ w446 w462]
                    frame Default {
                      n84 = Concatenate Strings("Framework error, it recieved \"" ("before match"), w441, "\" which is not expected." ("before match")) -> (w443:string)
                    }
                    frame "PostPostMsg" {
                      n85 = call "CSMP-PostPostMsg.vi"("State"=w456, "Args"=w455, "Source/target"=w454, "Pre-State In"=w453, "Pre-Args In"=w452, "Error In"=w460, "Session Error"=w446, "Module Name"=w458, "Response Arguments"=w457) -> ("State Out"=w447:string, "Args Out"=w448:string, "Source/target Out"=w449:string, "Pre-State Out"=w450:string, "Pre-Args Out"=w451:string, "Error"=w459:errorcluster)  [unwired: 5 in]
                    }
                    frame "PostSendMsg" {
                      n86 = call "CSMP-PostSendMsg.vi"("State"=w470, "Args"=w468, "Source/target"=w467, "Error In"=w464, "Session Error"=w462, "Module Name"=w471, "Response Arguments"=w461) -> ("State Out"=w469:string, "Args Out"=w466:string, "Source/target Out"=w465:string, "Error"=w463:errorcluster)  [unwired: 9 in]
                    }
                  }
                  n87 = call "_CSMObj-Unlock.vi"("Error In"=w418, "CSMQ In"=w419) -> ("error out"=w435:errorcluster, "CSMQ Out"=w432:T5)  [unwired: 8 in]
                }
                frame "", "<-" {
                  # "\"<-\"  : Added by Other JKI State Loop |  \"\" : Added by Current Loop"
                  n88 = Match Pattern(string=w477, regular expression="[\\t\\s]*>>>[\\t\\s]*") -> (before substring=w476:string, after substring=w479:string)  [unwired: 1 in, 2 out]
                  n89 = call "CSM - Convert Argument to Error.vi"("Argument"=w479) -> ("Error"=w475:errorcluster)  [unwired: 4 in]
                  n90 = case shown="\"macro: initialize\"" w491 {
                    selector: w491 -> [w501 w513 w523 w562 w570]
                    tunnel: w493 -> [w502 w506 w516 w560 w571]
                    tunnel: w497 -> [w503 w510 w526 w559 w566]
                    tunnel: w496 -> [w504 w509 w527 w558 w565]
                    tunnel: [w504 w509 w527 w558 w565] -> w495
                    tunnel: [w503 w510 w526 w559 w566] -> w494
                    tunnel: [w502 w507 w519 w560 w571] -> w492
                    tunnel: w490 -> [w500 w512 w520 w563 w569]
                    tunnel: [w501 w513 w522 w562 w570] -> w489
                    tunnel: [w500 w512 w521 w563 w569] -> w488
                    tunnel: [w499 w511 w525 w561 w568] -> w487
                    tunnel: w486 -> [w499 w511 w525 w561 w568]
                    tunnel: [w498 w508 w524 w564 w567] -> w485
                    tunnel: w484 -> [w498 w508 w524 w564 w567]
                    tunnel: w483 -> [_ _ _ _ _]
                    tunnel: [_ _ w515 _ _] -> w481
                    tunnel: w480 -> [_ _ w514 _ _]
                    frame Default {
                    }
                    frame "macro: initialize" {
                      n91 = call "Add State(s) to Queue__jkism.vi"("State(s) in Front (\"\")"="Macro: Initialize -><complete>" ("State(s) in Front (\"\")"), "State(s) in (\"\")"=w506) -> ("States Out"=w507:string)  [unwired: 13 in]
                    }
                    frame "macro: exit" {
                      w518 = "->[\\t\\s]*<[Ll][Oo]+[Pp]>[\\t\\s]*"  # -><loop>
                      # "if -><loop> is found, continous to parse next state"
                      # "#github 288 \nhttps://github.com/NEVSTOP-LAB/Communicable-State-Machine/issues/288\nWhen Macro: Exit is detected. CSM will stop LOOP firstly, then exit."
                      n92 = Match Pattern(string=w516, regular expression=w518) -> (offset past match=w517:i32)  [unwired: 1 in, 3 out]
                      n93 = Greater Or Equal To 0?(x=w517) -> (x >= 0?=w515:bool)
                      n94 = case shown="True" w515 {
                        tunnel: w523 -> [w530 _]
                        tunnel: [w530 _] -> w522
                        tunnel: [w529 _] -> w521
                        tunnel: w520 -> [w529 _]
                        tunnel: [w528 w543] -> w519
                        tunnel: w516 -> [w528 w533]
                        tunnel: w514 -> [_ w542]
                        frame False {
                        }
                        frame True {
                          w531 = "->[\\t\\s]*<[Ll][Oo]+[Pp]>[\\t\\s]*"  # -><loop>
                          w536 = "->[\\t\\s]*<[Ee][Nn][Dd]>[\\t\\s]*"  # -><end>
                          n95 = call "CSM - Break Down Multiple States String.vi"("States"=w533) -> ("Multiple States"=w534:string[])  [unwired: 10 in]
                          n96 = for {
                            tunnel: [w546] -> w535 mode=indexing if=w547
                            tunnel: w534 -> [w546] mode=indexing
                            tunnel: w531 -> [w544]
                            n97 = call "Remove Comments from Single-line.vi"("single-line text"=w546) -> ("single-line text without comments"=w545:string)  [unwired: 2 in]
                            n98 = Match Pattern(string=w545, regular expression=w544) -> (offset past match=w548:i32)  [unwired: 1 in, 3 out]
                            n99 = Less Than 0?(x=w548) -> (x < 0?=w547:bool)
                          }
                          n100 = call "CSM - Compact Multiple States.vi"("Multiple States"=w535) -> ("States"=w532:string)  [unwired: 9 in]
                          n101 = Match Pattern(string=w532, regular expression=w536) -> (before substring=w539:string, match substring=w540:string, after substring=w541:string, offset past match=w537:i32)  [unwired: 1 in]
                          n102 = Greater Or Equal To 0?(x=w537) -> (x >= 0?=w538:bool)
                          n103 = case shown="False" w538 {
                            tunnel: [w549 w555] -> w543
                            tunnel: w532 -> [w550 _]
                            tunnel: w539 -> [_ w557]
                            tunnel: w540 -> [_ w556]
                            tunnel: w541 -> [_ w552]
                            tunnel: w542 -> [w551 w553]
                            frame False {
                              n104 = call "Add State(s) to Queue__jkism.vi"("State(s) in Front (\"\")"=w551, "State(s) in (\"\")"=w550) -> ("States Out"=w549:string)  [unwired: 13 in]
                            }
                            frame True {
                              n105 = Concatenate Strings(w557, w556) -> (w554:string)
                              n106 = call "Add State(s) to Queue__jkism.vi"("State(s) in Front (\"\")"=w554, "State(s) in (\"\")"=w553, "State(s) at Back (\"\")"=w552) -> ("States Out"=w555:string)  [unwired: 12 in]
                            }
                          }
                        }
                      }
                    }
                    frame "exit" {
                    }
                    frame "async response" {
                    }
                  }
                }
                frame Default {
                  # "Error, should not be here."
                }
              }
              n107 = call "CSM - Convert Error to Argument.vi"("Error"=w130) -> ("Argument"=w129:string)  [unwired: 4 in]
              n108 = Select(t="Critical Error", s=w130, f=w161) -> (s? t:f=w157:string)
              n109 = Select(t=w129, s=w130, f=w160) -> (s? t:f=w159:string)
              n110 = Empty String/Path?(string/path=w153) -> (empty?=w168:bool)
              n111 = Empty String/Path?(string/path=w157) -> (empty?=w169:bool)
              n112 = Not(x=w168) -> (.not. x?=w167:bool)
              n113 = And(x=w169, y=w167) -> (x .and. y?=w154:bool)
            }
          }
        }
        n114 = Empty String/Path?(string/path=w83) -> (empty?=w82:bool)
        n115 = And(x=w82, y=w84) -> (x .and. y?=w85:bool)
      }
    }
    frame Error {
      # "Goto Error Handler State >>"
      # "preserve remaining states >>"
      n116 = call "_CSMObj-Log Error if in a Remote Session.vi"("Error"=w582, "Error In"=w585, "CSMQ In"=w586) -> ("CSMQ Out"=w581:T5)  [unwired: 7 in, 1 out]
      n117 = call "CSM - Convert Error to Argument.vi"("Error"=w582) -> ("Argument"=w587:string)  [unwired: 4 in]
    }
  }
  n118 = feedback-in #2(w6) -> ()
  n119 = feedback-in #3(w2) -> ()
  n120 = in-place {
    in-place-border: w31 -> [w602]
    in-place-border: [w598] -> w30
    in-place-border: w10 -> [w604]
    in-place-border: w2 -> [w613]
    in-place-border: w1 -> [w592]
    n121 = in-place-match #4(w36) -> (w606:string)
    n122 = in-place-match #5(w32) -> (w599:string)
    n123 = in-place-match #6(w44) -> (w611:string)
    n124 = in-place-match #7(w43) -> (w610:string)
    n125 = in-place-match #8(w41) -> (w607:string)
    n126 = in-place-match #9(w42) -> (w608:string)
    n127 = in-place-match #10(w27) -> (w609:string)
    n128 = Unbundle By Name(w602) -> ("Valid"=w612:bool)
    n129 = case shown="True" w612 {
      tunnel: w602 -> [w737 w756]
      tunnel: w611 -> [w746 w755]
      tunnel: [w746 w755] -> w593
      tunnel: w610 -> [w745 w754]
      tunnel: [w745 w754] -> w597
      tunnel: [w744 w753] -> w595
      tunnel: w608 -> [w744 w753]
      tunnel: [w743 w750] -> w596
      tunnel: w607 -> [w743 w750]
      tunnel: w599 -> [w742 w749]
      tunnel: [w742 w749] -> w600
      tunnel: [w741 w757] -> w605
      tunnel: w606 -> [w741 w757]
      tunnel: [T2 {"Name (\"\" to Use UUID)"="", "Current State"="", "Arguments"="", "Source Message"={"‘State"="", "’Arguments"="", "’Error"={"status"=FALSE, "code"=0, "source"=""}}, "Source Module"="", "Complete(T)/Start(F)"=FALSE, "LogType"=enum."State Change", "Time Stamp"=timestamp(0 s since 1904-01-01)} ("event data") w751] -> w598
      tunnel: [w740 w752] -> w594
      tunnel: w609 -> [w740 w752]
      tunnel: w604 -> [w738 w748]
      tunnel: [w738 w748] -> w603
      tunnel: [w737 w747] -> w601
      frame False {
      }
      frame True {
        n130 = call "GEvt-Generate State Change Log.vi"("CSM Global Log Event"=w756, "Current State"=w755, "Arguments"=w754, "Source Message.*State"=w753, "Source Message.*Arguments"=w752, "Source Module"=w750, "Name (\"\" to Use UUID)"=w749, "CSM:LogFilter.lvclass"=w748) -> ("CSM Global Log Event Out"=w747:T4, "Event Data"=w751:T2)  [unwired: 10 in]
      }
    }
    n131 = call "Auto Broadcast State.vi"("CSM Name"=w600, "Current State"=w593, "States Queue"=w605) -> ("Remaining States Queue"=w614:string)  [unwired: 6 in]
    n132 = case shown="\"Critical Error\", \"Exit\"" w593 {
      tunnel: [w617 w640] -> w616
      tunnel: [w618 w639] -> w615
      tunnel: w614 -> [w618 w636]
      tunnel: w613 -> [_ w632]
      tunnel: w603 -> [_ w622]
      tunnel: w601 -> [_ w620]
      tunnel: w600 -> [w617 w621]
      tunnel: w592 -> [_ w630]
      frame "False", Default {
      }
      frame "Critical Error", "Exit" {
        # "#github\nmove it here to release registration when\ncritical error occured."
        # "#github \nThis is used to process:\n1. Sync/Async message of \"Macro: Exit\",\"Exit\",\"Critical Error\"\n2. State registration of \"Macro: Exit\",\"Exit\",\"Critical Error\""
        n133 = call "_CSMObj-Unregister Internal Registry Rules.vi"("CSM:LogFilter.lvclass"=w622, "Name (\"\" to Use UUID)"=w621, "CSM Global Log Event"=w620, "CSMQ In"=w630) -> ("error out"=w624:errorcluster, "CSMQ Out"=w626:T5)  [unwired: 6 in]
        n134 = call "_CSMObj-Lock State.vi"("Error In"=w624, "CSMQ In"=w626) -> ("error out"=w625:errorcluster, "CSMQ Out"=w623:T5, "Error"=w629:errorcluster)  [unwired: 5 in, 1 out]
        n135 = call "_CSMObj-Unlock.vi"("Error In"=w625, "CSMQ In"=w623) -> ("error out"=w627:errorcluster, "CSMQ Out"=w628:T5)  [unwired: 8 in]
        n136 = call "Parse Action State After Exit.vi"("States"=w636) -> ("Need to Process"=w631:string, "Remaining States"=w637:string)  [unwired: 9 in]
        n137 = call "_CSMOFGV Release.vi"("Error In"=w627, "CSMQ"=w628) -> ("error out"=w619:errorcluster)  [unwired: 9 in]
        n138 = case shown="Default" w631 {
          selector: w631 -> [_ w646]
          tunnel: w621 -> [w643 w653]
          tunnel: w620 -> [w642 w652]
          tunnel: [w643 w651] -> w633
          tunnel: [w642 w650] -> w634
          tunnel: w622 -> [w641 w649]
          tunnel: [w641 w648] -> w635
          tunnel: w632 -> [_ w647]
          tunnel: w629 -> [_ w644]
          tunnel: w619 -> [_ _]
          frame "" {
          }
          frame Default {
            n139 = call "CSM - Break Down Multiple States String.vi"("States"=w646) -> ("Multiple States"=w645:string[])  [unwired: 10 in]
            n140 = for "While current line is a comment and there are more lines to process" {
              shift-right: [w658] -> w651
              shift-left: w653 -> [w670]
              shift-right: [w656] -> w650
              shift-left: w652 -> [w669]
              shift-right: [w657] -> w648
              shift-left: w649 -> [w659]
              tunnel: w647 -> [w660]
              tunnel: w645 -> [w655] mode=indexing
              tunnel: w644 -> [w654]
              # "source/target"
              # "Pre-Args"
              # "Pre-State"
              # "name"
              # "remaining lines"
              # "args"
              # "state"
              n141 = call "Remove Comments from Single-line.vi"("single-line text"=w655) -> ("single-line text without comments"=w668:string)  [unwired: 2 in]
              n142 = call "Split Single-line Message.vi"("single-line text"=w668) -> ("operator"=w665:string, "state"=w666:string, "args"=w667:string, "source/target"=w664:string)  [unwired: 6 in]
              n143 = call "Split Single-line Reason Parts.vi"("Single-line -& Reason"=w664) -> ("CSM Name"=w663:string, "`State"=w662:string, "`Arguments"=w661:string)  [unwired: 12 in]
              n144 = case shown="\"-&\"" w665 {
                selector: w665 -> [w677 _ _]
                tunnel: w666 -> [w680 w710 _]
                tunnel: w667 -> [w679 w711 _]
                tunnel: w670 -> [w678 w708 w727]
                tunnel: w663 -> [w681 w707 _]
                tunnel: w669 -> [w676 w709 w728]
                tunnel: [w675 w709 w728] -> w656
                tunnel: [w674 w708 w727] -> w658
                tunnel: w662 -> [_ w706 _]
                tunnel: w661 -> [_ w705 _]
                tunnel: w659 -> [w673 w704 w726]
                tunnel: w660 -> [w672 _ _]
                tunnel: [w671 w704 w726] -> w657
                tunnel: w654 -> [_ w703 _]
                frame "->", "->|" {
                  # "Async Call and post message to other loop"
                  n145 = case shown="\"<state>\"" w681 {
                    selector: w681 -> [_ w687]
                    tunnel: w680 -> [_ w693]
                    tunnel: w679 -> [_ w691]
                    tunnel: w678 -> [w683 w692]
                    tunnel: w677 -> [_ _]
                    tunnel: [w684 w694] -> w675
                    tunnel: w676 -> [w684 w695]
                    tunnel: [w683 w692] -> w674
                    tunnel: w673 -> [w682 w686]
                    tunnel: w672 -> [_ w688]
                    tunnel: [w682 w686] -> w671
                    frame Default {
                    }
                    frame "<state>" {
                      n146 = call "Replace LastResp Token.vi"("LastResp"="" ("Response Before \"Error Handler\""), "Argument"=w691) -> ("Argument Out"=w689:string)  [unwired: 5 in]
                      n147 = call "GEvt-Generate Status Log.vi"("CSM Global Log Event"=w695, "Current State"=w693, "Arguments"=w689, "Source Module"=w687, "Name (\"\" to Use UUID)"=w692, "CSM:LogFilter.lvclass"=w686) -> ("CSM Global Log Event Out"=w694:T4)  [unwired: 12 in, 1 out]
                      n148 = call "Cache-StatusChangeEventRef.vi"("Name (\"\" to Use UUID) In"=w692) -> ("Status Change Event"=w696:refnum<user-event>)  [unwired: 9 in, 1 out]
                      n149 = Bundle(cluster=T11 {"ModuleName"="", "Status"="", "Arguments"=""} ("event data"), "ModuleName"=w692, "Status"=w693, "Arguments"=w689) -> (w697:T11)
                      n150 = Not A Number/Path/Refnum?(number/path/refnum=w696) -> (NaN/Path/Refnum?=w699:bool)
                      n151 = case shown="False" w699 {
                        tunnel: w696 -> [w701 _]
                        tunnel: w697 -> [w700 _]
                        frame False {
                          n152 = Generate User Event(user event=w701, event data cluster=w700) -> ()  [unwired: 2 in, 2 out]
                        }
                        frame True {
                        }
                      }
                      n153 = call "CSMP-Broadcast.vi"("State"=w693, "Args"=w689, "Source/target"=w687, "Response For Message.’Error"=w688, "Module Name"=w692, "Msg Type"=_CSM_MSG_TYPE."Broadcast(-><state>)") -> ()  [unwired: 8 in, 6 out]
                    }
                  }
                }
                frame "-&" {
                  # "Synchonized Call send msg and wait response"
                  n154 = case shown="\"PostSendMsg\"" w710 {
                    selector: w710 -> [_ w717 w724]
                    tunnel: w707 -> [_ w715 w722]
                    tunnel: w711 -> [_ w716 w723]
                    tunnel: "" ("Response Before \"Error Handler\"") -> [_ w718 w720]
                    tunnel: w708 -> [_ w719 w725]
                    tunnel: w706 -> [_ w714 _]
                    tunnel: w705 -> [_ w713 _]
                    tunnel: w703 -> [_ w712 w721]
                    frame Default {
                    }
                    frame "PostPostMsg" {
                      n155 = call "CSMP-PostPostMsg.vi"("State"=w717, "Args"=w716, "Source/target"=w715, "Pre-State In"=w714, "Pre-Args In"=w713, "Session Error"=w712, "Module Name"=w719, "Response Arguments"=w718) -> ()  [unwired: 6 in, 6 out]
                    }
                    frame "PostSendMsg" {
                      n156 = call "CSMP-PostSendMsg.vi"("State"=w724, "Args"=w723, "Source/target"=w722, "Session Error"=w721, "Module Name"=w725, "Response Arguments"=w720) -> ()  [unwired: 10 in, 4 out]
                    }
                  }
                }
                frame Default {
                  # "Error, should not be here."
                }
              }
            }
          }
        }
        n157 = Unbundle By Name(w634) -> ("Valid"=w638:bool)
        n158 = case shown="False" w638 {
          tunnel: w634 -> [_ w732]
          tunnel: w633 -> [w730 w734]
          tunnel: [w730 w734] -> w640
          tunnel: [w729 w736] -> w639
          tunnel: w637 -> [w729 w736]
          tunnel: w635 -> [_ w733]
          frame False {
          }
          frame True {
            w731 = TRUE ("Enable?")
            n159 = call "GEvt-Generate Remaining States Log.vi"("CSM Global Log Event"=w732, "Remaining States"=w736, "Name (\"\" to Use UUID)"=w734, "Enable?"=w731, "CSM:LogFilter.lvclass"=w733) -> ("CSM Global Log Event Out"=w735:T4)  [unwired: 13 in, 1 out]
            n160 = call "GEvt-Generate Module Destroyed Log.vi"("CSM Global Log Event"=w735, "Name (\"\" to Use UUID)"=w734, "Enable?"=w731, "CSM:LogFilter.lvclass"=w733) -> ()  [unwired: 14 in, 2 out]
          }
        }
      }
    }
    n161 = in-place-match #4(w615) -> (→"Remaining States":string)
    n162 = in-place-match #5(w616) -> (→"Name Used":string)
    n163 = in-place-match #6(w593) -> (→"Current State":string)
    n164 = in-place-match #7(w597) -> (→"Arguments":string)
    n165 = in-place-match #8(w596) -> (→">> Source CSM >>":string)
    n166 = in-place-match #9(w595) -> (w29:string)
    n167 = in-place-match #10(w594) -> (w26:string)
  }
  n168 = feedback-in #1(w30) -> ()
  n169 = Bundle By Name(cluster=T1 {"‘State"="", "’Arguments"="", "’Error"={"status"=FALSE, "code"=0, "source"=""}} (">> Response Source Message >>"), "‘State"=w29, "’Arguments"=w26, "’Error"=w21) -> (→">> Response Source Message >>":T1)
